vi "LoginGui.vi"() -> (3 "ok?":bool)   [LabVIEW 2016]
uses:
  LoginGui.Action.ctl
  Tools/Config/Config.Global.vi
panel:
  out "_loop":i32(ring)=4
  in  "pwd_Password":string caption="Password"
  in  "CancelButton":bool
  in  "OKButton":bool
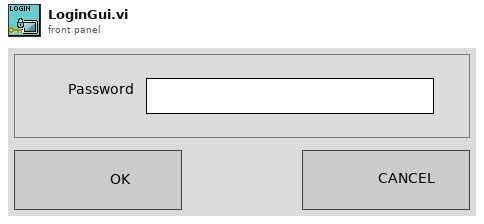
[diagram p1: front panel]
types:
  T1 = typedef "LoginGui.Action.ctl" = enum32{"idle", "constructor", "destructor", "--- Login GUI ---"}
  T2 = enum8{"Enabled", "Disabled", "Disabled and Grayed Out"}
  T3 = typedef "LVPositionTypeDef.ctl" = cluster{"Left":i32, "Top":i32}
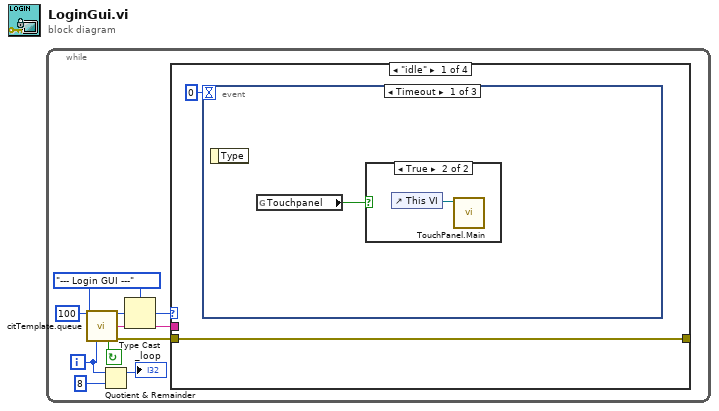
[diagram p0: block diagram]
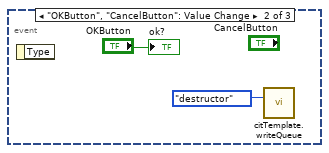
[diagram p3: hidden frame]
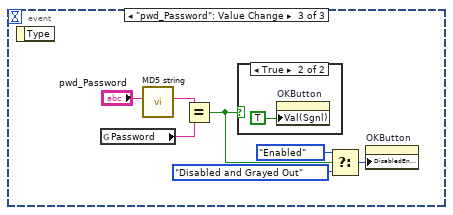
[diagram p4: hidden frame]
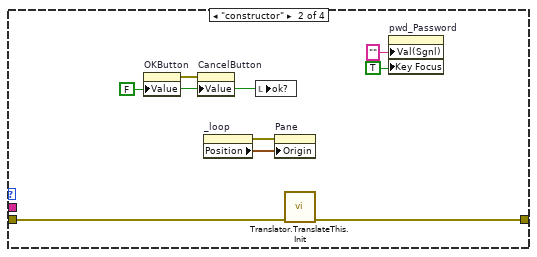
[diagram p6: hidden frame]
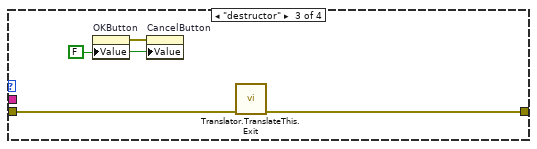
[diagram p7: hidden frame]
diagram:
  n1 = while {
    i -> [w1]
    stop <- w7 continue-if-true
    w6 = LoginGui.Action."--- Login GUI ---" ("Action")
    n2 = call "citTemplate.queue.vi"("ms timeout (250 ms)"=100, "event enum"=w6, "iteration (-1)"=w1) -> ("event out"=w10:u32, "(flatten) data out"=w9:string, "continue"=w7:bool, "error out"=w8:errorcluster)  [unwired: 2 in, 7 out]
    n3 = Quotient & Remainder(x=w1, y=8) -> (x-y*floor(x/y)=→"_loop":i32)  [unwired: 1 out]
    n4 = Type Cast(type=w6, x=w10) -> (*(type *) &x=w5:T1)
    n5 = case shown="\"idle\"" w5 {
      tunnel: w9 -> [_ _ _ _]
      tunnel: w8 -> [w11 w28 w34 w37]
      tunnel: [w11 w27 w33 w37] -> _
      frame "idle" {
        n6 = event shown="[0] Timeout" {
          selector: _ -> [_ _ _]
          dyn-events: _ -> [_ _ _]
          timeout: 0 -> [_ _ _]
          event Timeout {
            n7 = event-data() -> ()  [unwired: 1 in, 1 out]
            n8 = global read "Config.Global.vi" "Touchpanel"() -> (w13:bool)
            n9 = case shown="True" w13 {
              frame False {
              }
              frame True {
                n10 = control-ref of="This VI"() -> (w14:refnum<vi>)
                n11 = call "TouchPanel.Main.vi"("VI ref"=w14) -> ()  [unwired: 9 in, 2 out]
              }
            }
          }
          event "OKButton", "CancelButton": Value Change {
            n12 = event-data() -> ()  [unwired: 1 in, 1 out]
            n13 = call "citTemplate.writeQueue.vi"("event in (if not connected:all statemachine with data event)"=LoginGui.Action."destructor" ("Action")) -> ()  [unwired: 14 in, 1 out]
            "ok?" <- "OKButton"
          }
          event "pwd_Password": Value Change {
            n14 = event-data() -> ()  [unwired: 1 in, 1 out]
            n15 = global read "Config.Global.vi" "Password"() -> (w19:string)
            n16 = call "MD5 string.vi"("Message String"="pwd_Password") -> ("MD5 message-digest"=w18:string)  [unwired: 10 in]
            n17 = Equal?(x=w18, y=w19) -> (x = y?=w17:bool)
            n18 = case shown="True" w17 {
              frame False {
              }
              frame True {
                n19 = property on="OKButton" class="Bool (strict)"("Val(Sgnl)"=TRUE ("Value (Signaling)")) -> ()  [unwired: 2 in, 2 out]
              }
            }
            n20 = Select(t=T2."Enabled" ("Disabled"), s=w17, f=T2."Disabled and Grayed Out" ("Disabled")) -> (s? t:f=w22:T2)
            n21 = property on="OKButton" class="Bool (strict)"("DisabledEnum"=w22) -> ()  [unwired: 2 in, 2 out]
          }
        }
      }
      frame "constructor" {
        w31 = FALSE ("_b_OK")
        n22 = property on="OKButton" class="Bool (strict)"("Value"=w31) -> (error out=w32:errorcluster)  [unwired: 2 in, 1 out]
        n23 = property on="CancelButton" class="Bool (strict)"(error in=w32, "Value"=w31) -> ()  [unwired: 1 in, 2 out]
        n24 = property on="_loop" class="Ring (strict)"() -> (error out=w29:errorcluster, "Position"=w30:T3)  [unwired: 2 in, 1 out]
        n25 = local write "ok?"(w31) -> ()
        n26 = property on="Pane" class="Pane"(error in=w29, "Origin"=w30) -> ()  [unwired: 1 in, 2 out]
        n27 = call "Translator.TranslateThis.Init.vi"("error in"=w28) -> ("error out"=w27:errorcluster)  [unwired: 10 in]
        n28 = property on="pwd_Password" class="Str"("Val(Sgnl)"="" ("Password"), "Key Focus"=TRUE) -> ()  [unwired: 2 in, 2 out]
      }
      frame "destructor" {
        w35 = FALSE ("_b_OK")
        n29 = property on="OKButton" class="Bool (strict)"("Value"=w35) -> (error out=w36:errorcluster)  [unwired: 2 in, 1 out]
        n30 = property on="CancelButton" class="Bool (strict)"(error in=w36, "Value"=w35) -> ()  [unwired: 1 in, 2 out]
        n31 = call "Translator.TranslateThis.Exit.vi"("error in"=w34) -> ("error out"=w33:errorcluster)  [unwired: 10 in]
      }
      frame "--- Login GUI ---" {
      }
    }
  }
